vi "Get_Variant_Array_Size.vi"(8 "error in (no error)":errorcluster, 11 "Array in":variant) -> (0 "error out":errorcluster, 1 "Size(s)":u32[](array[numeric]), 2 "N dims":u32, 3 "Array out":variant)   [LabVIEW 2012]
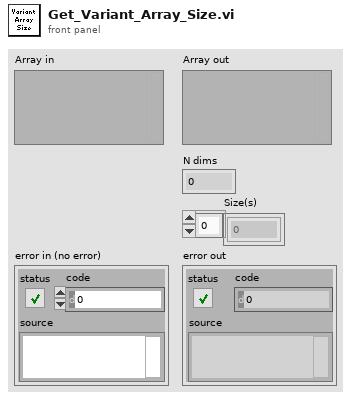
[diagram p1: front panel]
types:
  T1 = cluster{"length":u16, "private":u8, "type":enum8{"<Null>", "I8", "I16", "I32", "I64", "U8", "U16", "U32", "U64", "SGL", "DBL", "EXT", "CSG", "CDB", "CXT", "0x0F", "0x10", "0x11", "0x12", "0x13", "0x14", "Enum U8", "Enum U16", "Enum U32", "Enum U64", "SGL PQ", "DBL PQ", "EXT PQ", "CSG PQ", "CDB PQ", "CXT PQ", "0x1F", "0x20", "Boolean", "0x22", "0x23", "0x24", "0x25", "0x26", "0x27", "0x28", "0x29", "0x2A", "0x2B", "0x2C", "0x2D", "0x2E", "0x2F", "String", "0x31", "Path", "Pict", "0x34", "0x35", "0x36", "DAQ", "0x38", "0x39", "0x3A", "0x3B", "0x3C", "0x3D", "0x3E", "0x3F", "Array", "0x41", "0x42", "0x43", "0x44", "0x45", "0x46", "0x47", "0x48", "0x49", "0x4A", "0x4B", "0x4C", "0x4D", "0x4E", "0x4F", "Cluster", "0x51", "0x52", "Variant", "Waveform", "0x55", "0x56", "0x57", "0x58", "0x59", "0x5A", "0x5B", "0x5C", "0x5D", "0x5E", "0x5F", "0x60", "0x61", "0x62", "0x63", "0x64", "0x65", "0x66", "0x67", "0x68", "0x69", "0x6A", "0x6B", "0x6C", "0x6D", "0x6E", "0x6F", "Refnum"}, "# elements":u16}
  T2 = enum8{"<Null>", "I8", "I16", "I32", "I64", "U8", "U16", "U32", "U64", "SGL", "DBL", "EXT", "CSG", "CDB", "CXT", "0x0F", "0x10", "0x11", "0x12", "0x13", "0x14", "Enum U8", "Enum U16", "Enum U32", "Enum U64", "SGL PQ", "DBL PQ", "EXT PQ", "CSG PQ", "CDB PQ", "CXT PQ", "0x1F", "0x20", "Boolean", "0x22", "0x23", "0x24", "0x25", "0x26", "0x27", "0x28", "0x29", "0x2A", "0x2B", "0x2C", "0x2D", "0x2E", "0x2F", "String", "0x31", "Path", "Pict", "0x34", "0x35", "0x36", "DAQ", "0x38", "0x39", "0x3A", "0x3B", "0x3C", "0x3D", "0x3E", "0x3F", "Array", "0x41", "0x42", "0x43", "0x44", "0x45", "0x46", "0x47", "0x48", "0x49", "0x4A", "0x4B", "0x4C", "0x4D", "0x4E", "0x4F", "Cluster", "0x51", "0x52", "Variant", "Waveform", "0x55", "0x56", "0x57", "0x58", "0x59", "0x5A", "0x5B", "0x5C", "0x5D", "0x5E", "0x5F", "0x60", "0x61", "0x62", "0x63", "0x64", "0x65", "0x66", "0x67", "0x68", "0x69", "0x6A", "0x6B", "0x6C", "0x6D", "0x6E", "0x6F", "Refnum"}
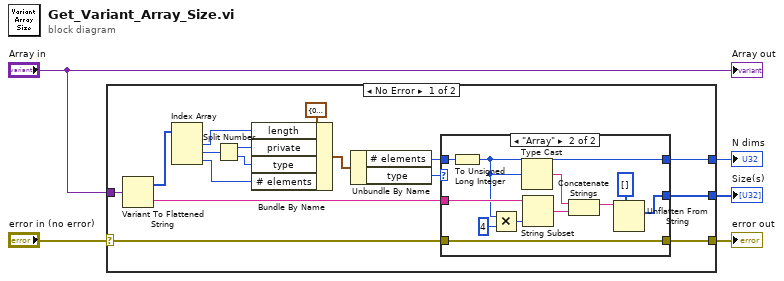
[diagram p0: block diagram]
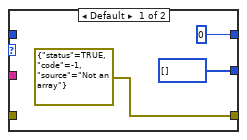
[diagram p2: hidden frame]
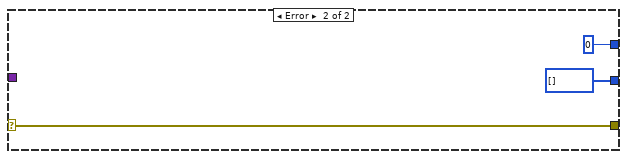
[diagram p3: hidden frame]
diagram:
  n1 = case shown="No Error" "error in (no error)" {
    selector: "error in (no error)" -> [w7 w38]
    tunnel: [w6 w38] -> w3
    tunnel: [w21 u32 0] -> w2
    tunnel: [w20 u32[] [] ("Size(s)")] -> w1
    tunnel: "Array in" -> [w16 _]
    frame No Error {
      n2 = Variant To Flattened String(Variant=w16) -> (data string=w17:string, 1:w9:i16[])
      n3 = Index Array(array=w9) -> (element #1=w14:i16, element #2=w11:i16, element #3=w10:i16)  [unwired: 3 in]
      n4 = Split Number(x=w11) -> (hi(x)=w13:u8, lo(x)=w12:u8)
      n5 = Bundle By Name(cluster=T1 {"length"=0, "private"=0, "type"=enum."<Null>", "# elements"=0} ("Type Descriptor Header"), "length"=w14, "private"=w13, "type"=w12, "# elements"=w10) -> (w8:T1)
      n6 = Unbundle By Name(w8) -> ("# elements"=w18:u16, "type"=w19:T2)
      n7 = case shown="\"Array\"" w19 {
        tunnel: w17 -> [_ w29]
        tunnel: [u32 0 w26] -> w21
        tunnel: [u32[] [] ("Size(s)") w28] -> w20
        tunnel: w18 -> [_ w27]
        tunnel: w7 -> [_ w25]
        tunnel: [errorcluster {"status"=TRUE, "code"=-1, "source"="Not an array"} ("error out") w25] -> w6
        frame Default {
        }
        frame "Array" {
          n8 = To Unsigned Long Integer(number=w27) -> (unsigned 32bit integer=w26:u32)
          n9 = Multiply(x=w26, y=u32 4) -> (x*y=w33:u32)
          n10 = Type Cast(x=w26) -> (*(type *) &x=w30:string)  [unwired: 1 in]
          n11 = String Subset(string=w29, length (rest)=w33) -> (substring=w31:string)  [unwired: 1 in]
          n12 = Concatenate Strings(w30, w31) -> (w32:string)
          n13 = Unflatten From String(type=u32[] [] ("Size(s)"), binary string=w32) -> (value=w28:u32[])  [unwired: 3 in, 2 out]
        }
      }
    }
    frame Error {
    }
  }
  "error out" <- w3
  "N dims" <- w2
  "Size(s)" <- w1
  "Array out" <- "Array in"
